vi "Periodic Tasks.vi"(8 "error in":errorcluster) -> ()   [LabVIEW 2016]
doc: "This VI runs in parallel to other tasks. It can contain as many user-defined periodic loops as you need. These can carry out PID or other sorts of timed response."
uses:
  <vilib>/Rock Robotics/WPI/Utilities/WPI_GetSetVariantRefNum.vi
panel:
  out "Object 2":T1
  out "Data Out":u8[](array[numeric])
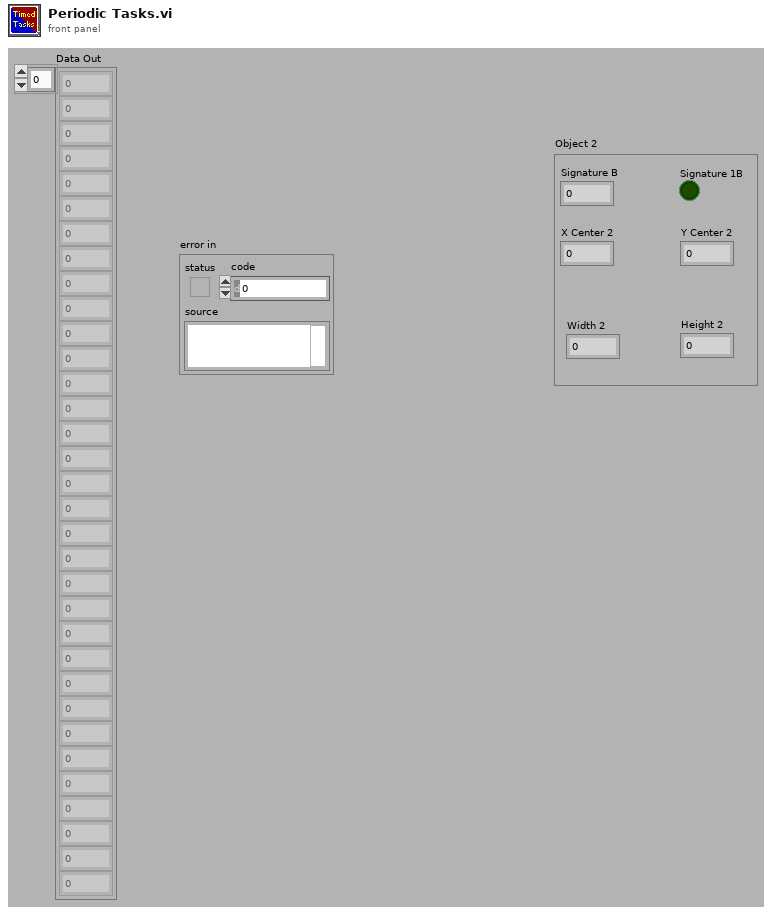
[diagram p1: front panel]
types:
  T1 = cluster{"Signature B":dbl, "Signature 1B":bool, "X Center 2":dbl, "Y Center 2":dbl, "Width 2":dbl, "Height 2":dbl}
  T2 = typedef "WPI_I2CDevRef.ctl" = cluster{"DevStatus":errorcluster, "Device Address":u8, "Handle":i32, "I2C Bus":T3}
  T3 = typedef "i2c_bus.ctl" = enum16{"I2C On-Board", "I2C MXP", "Invalid"}
  T4 = typedef "WPI_JoystickDevRef.ctl" = cluster{"Device":T5}
  T5 = typedef "WPI_JoystickDeviceEnum.ctl" = enum16{"USB 0", "USB 1", "USB 2", "USB 3", "USB 4", "USB 5"}
  T6 = typedef "WPI_MotorControlDeviceRef.ctl" = cluster{"DeviceStatus":errorcluster, "Type":T7, "PWM":cluster{"PWM Channel":T8, "DeadBand":T9}, "CAN":cluster{"Device Number":u8, "SetOutput VI Ref":variant, "GetOutput VI Ref":variant, "Enable VI Ref":variant, "Disable VI Ref":variant, "Data":variant}, "Invert":bool}
  T7 = typedef "WPI_MotorControlType.ctl" = enum16{"PWM", "CAN"}
  T8 = typedef "FPGA_DIOPWMChannel.ctl" = enum8{"PWM 0", "PWM 1", "PWM 2", "PWM 3", "PWM 4", "PWM 5", "PWM 6", "PWM 7", "PWM 8", "PWM 9", "PWM MXP 0", "PWM MXP 1", "PWM MXP 2", "PWM MXP 3", "PWM MXP 4", "PWM MXP 5", "PWM MXP 6", "PWM MXP 7", "PWM MXP 8", "PWM MXP 9", "Invalid"}
  T9 = typedef "WPI_PWMDeadband.ctl" = cluster{"Name":string, "maxPositivePwm":i32, "minPositivePwm":i32, "centerPwm":i32, "maxNegativePwm":i32, "minNegativePwm":i32, "angularRange":u16}
  T10 = cluster{"Height":dbl, "Signature A":dbl, "Signature 1A":bool, "X Center":dbl, "Y Center":dbl, "Width":dbl}
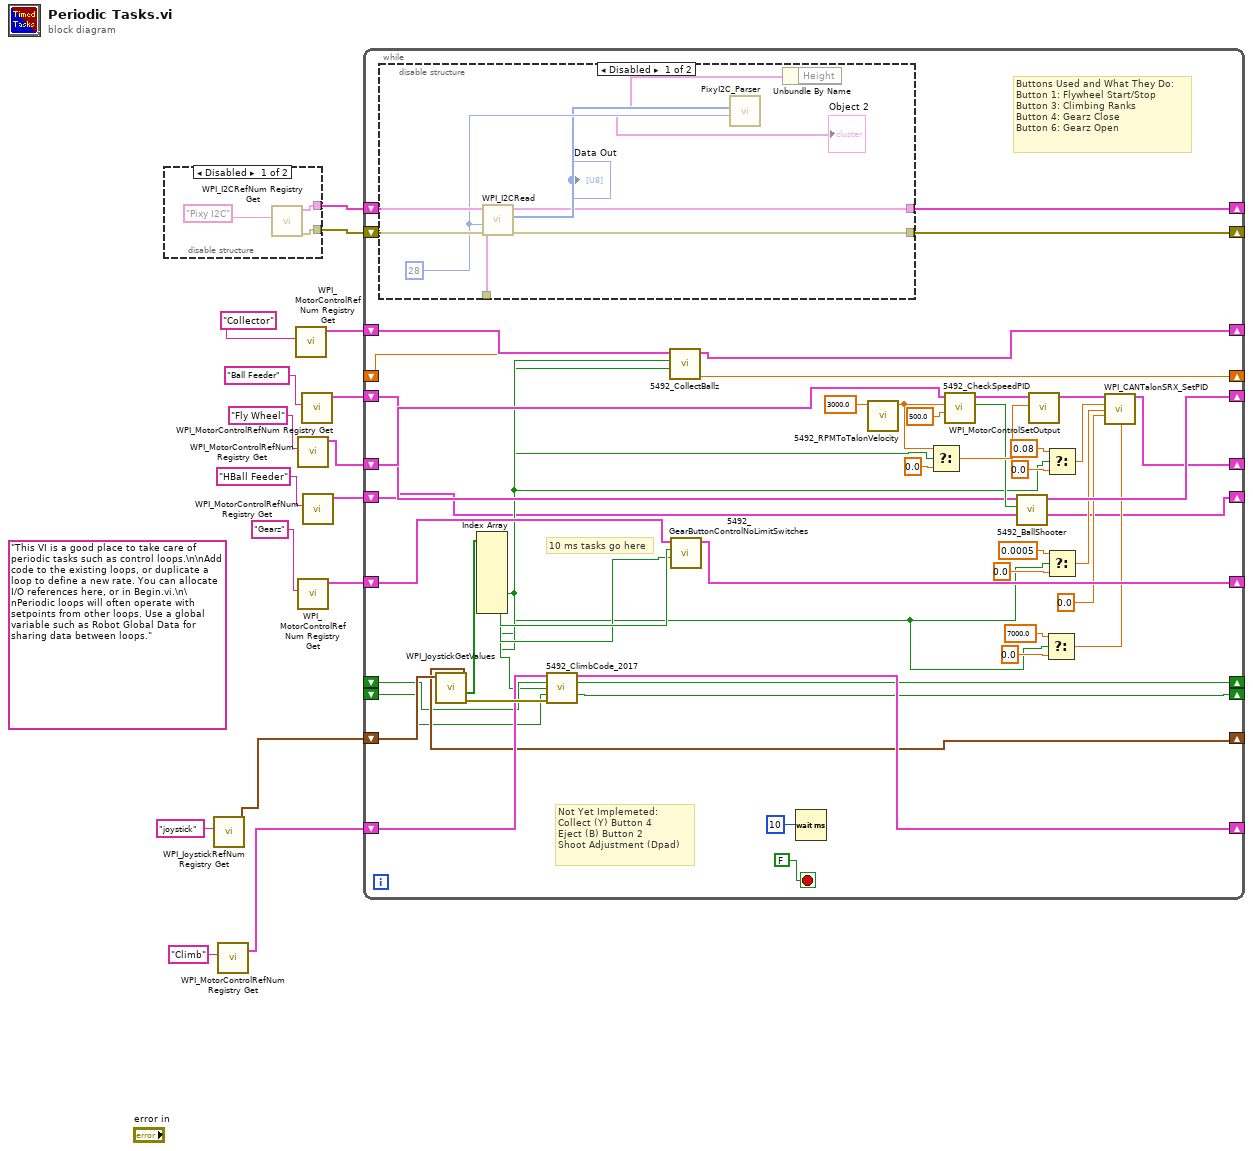
[diagram p0: block diagram]
diagram:
  (unwired) "This VI is a good place to take care of periodic tasks such as control loops.\n\nAdd code to the existing loops, or duplicate a loop to define a new rate. You can allocate I/O references here, or in Begin.vi.\n\nPeriodic loops will often operate with setpoints from other loops. Use a global variable such as Robot Global Data for sharing data between loops."
  n1 = disable-structure shown="Disabled" {
    disable-tunnel: [w18 _] -> w6
    disable-tunnel: [w17 _] -> w5
    frame Disabled {
      n2 = call <vilib>:"WPI_I2CRefNum Registry Get.vi"("refnum name"="Pixy I2C") -> ("error out"=w17:errorcluster, "I2CDevRef"=w18:T2)  [unwired: 9 in]
    }
    frame Enabled {
    }
  }
  n3 = call <vilib>:"WPI_JoystickRefNum Registry Get.vi"("refnum name"="joystick") -> ("JoystickDevRef"=w14:T4)  [unwired: 9 in, 1 out]
  n4 = call <vilib>:"WPI_MotorControlRefNum Registry Get.vi"("refnum name"="Climb") -> ("MotorControlDevRef"=w13:T6)  [unwired: 9 in, 1 out]
  n5 = call <vilib>:"WPI_MotorControlRefNum Registry Get.vi"("refnum name"="Collector") -> ("MotorControlDevRef"=w3:T6)  [unwired: 9 in, 1 out]
  n6 = call <vilib>:"WPI_MotorControlRefNum Registry Get.vi"("refnum name"="Fly Wheel") -> ("MotorControlDevRef"=w9:T6)  [unwired: 9 in, 1 out]
  n7 = call <vilib>:"WPI_MotorControlRefNum Registry Get.vi"("refnum name"="Gearz") -> ("MotorControlDevRef"=w11:T6)  [unwired: 9 in, 1 out]
  n8 = call <vilib>:"WPI_MotorControlRefNum Registry Get.vi"("refnum name"="Ball Feeder") -> ("MotorControlDevRef"=w7:T6)  [unwired: 9 in, 1 out]
  n9 = call <vilib>:"WPI_MotorControlRefNum Registry Get.vi"("refnum name"="HBall Feeder") -> ("MotorControlDevRef"=w1:T6)  [unwired: 9 in, 1 out]
  n10 = while {
    shift-right: [w65] -> _
    shift-left: w13 -> [w66]
    shift-right: [w64] -> _
    shift-left: w14 -> [w69]
    shift-right: [w62] -> _
    shift-left: w11 -> [w63]
    shift-right: [w39] -> _
    shift-left: w9 -> [w60]
    shift-right: [w53] -> _
    shift-left: w7 -> [w54]
    shift-right: [w52] -> _
    shift-left: _ -> [w51]
    shift-right: [w50] -> _
    shift-left: _ -> [w49]
    shift-right: [w45] -> _
    shift-left: w5 -> [w47]
    shift-right: [w46] -> _
    shift-left: w6 -> [w48]
    shift-right: [w37] -> _
    shift-left: w3 -> [w38]
    shift-right: [w34] -> _
    shift-left: _ -> [w33]
    shift-right: [w20] -> _
    shift-left: w1 -> [w21]
    stop <- FALSE stop-if-true
    # "Not Yet Implemeted:\nCollect (Y) Button 4\nEject (B) Button 2\nShoot Adjustment (Dpad)"
    # "Buttons Used and What They Do:\nButton 1: Flywheel Start/Stop\nButton 3: Climbing Ranks\nButton 4: Gearz Close\nButton 6: Gearz Open"
    # "10 ms tasks go here"
    n11 = disable-structure shown="Disabled" {
      disable-tunnel: w48 -> [w76 _]
      disable-tunnel: w47 -> [w75 _]
      disable-tunnel: [w74 _] -> w46
      disable-tunnel: [w73 _] -> w45
      frame Disabled {
        w79 = u8 28 ("I2CBytesToRead")
        n12 = call <vilib>:"WPI_I2CRead.vi"("error in (no error)"=w75, "I2CBytesToRead"=w79, "I2CDevRef"=w76) -> ("error out"=w73:errorcluster, "Data Out"=w78:u8[], "I2CDevRef"=w74:T2)  [unwired: 6 in]
        "Data Out" <- w78
        n13 = call "PixyI2C_Parser.vi"("Array Size"=w79, "Array"=w78) -> ("Object 2"=→"Object 2":T1, "Object 1"=w72:T10)  [unwired: 7 in]
        n14 = Unbundle By Name(w72) -> ()  [unwired: 1 out]
      }
      frame Enabled {
      }
    }
    n15 = call <vilib>:"WPI_JoystickGetValues.vi"("JoystickDevRef"=w69) -> ("error out"=w67:errorcluster, "Buttons"=w68:bool[], "JoystickDevRef"=w64:T4)  [unwired: 6 in, 2 out]
    n16 = Index Array(array=w68) -> (element #1=w44:bool, element #2=w35:bool, element #3=w43:bool, element #4=w36:bool, element #5=w42:bool, element #6=w29:bool)  [unwired: 8 in, 2 out]
    n17 = call "5492_ClimbCode_2017.vi"("MotorControlDevRef"=w66, "Stuck? (Input)"=w51, "Button Press"=w42, "Rope Grabbed? (Input)"=w49, "error in (no error)"=w67) -> ("MotorControlDevRef"=w65:T6, "Stuck? (Output)"=w52:bool, "Rope Grabbed? (Output)"=w50:bool)  [unwired: 7 in, 1 out]
    n18 = call "5492_CollectBallz.vi"("Current Collect"=w33, "Reject Ballz"=w35, "Collect Ballz"=w36, "MotorControlDevRef"=w38) -> ("Current Collect"=w34:dbl, "MotorControlDevRef"=w37:T6)  [unwired: 6 in]
    n19 = call "5492_GearButtonControlNoLimitSwitches.vi"("Button (Close)"=w43, "Button (Open)"=w44, "MotorControlDevRef"=w63) -> ("MotorControlDevRef"=w62:T6)  [unwired: 8 in]
    n20 = Wait (ms)(milliseconds to wait=u32 10) -> ()  [unwired: 1 out]
    n21 = call "5492_RPMToTalonVelocity.vi"("RPM"=3000.0) -> ("Talon Velocity"=w56:dbl)  [unwired: 10 in]
    n22 = Select(t=w56, s=w29, f=0.0) -> (s? t:f=w58:dbl)
    n23 = call "5492_CheckSpeedPID.vi"("Margin Of Error"=500.0, "Goal"=w56, "CAN Talon SRX Ref In"=w60) -> ("Speed Reached"=w55:bool, "CAN Talon SRX Ref In Out"=w59:T6)  [unwired: 6 in]
    n24 = call "5492_BallShooter.vi"("MotorControlDevRef Horizontal"=w21, "Shoot?"=w55, "MotorControlDevRef In"=w54) -> ("MotorControlDevRef Horizontal Out"=w20:T6, "MotorControlDevRef Out"=w53:T6)  [unwired: 7 in]
    n25 = call <vilib>:"WPI_MotorControlSetOutput.vi"("Output"=w58, "MotorControlDevRef"=w59) -> ("MotorControlDevRef"=w40:T6)  [unwired: 7 in, 2 out]
    n26 = Select(t=7000.0, s=w29, f=0.0) -> (s? t:f=w25:dbl)
    n27 = Select(t=0.08 ("f"), s=w29, f=0.0) -> (s? t:f=w28:dbl)
    n28 = Select(t=0.0005 ("f"), s=w29, f=0.0) -> (s? t:f=w27:dbl)
    n29 = call <vilib>:"WPI_CANTalonSRX_SetPID.vi"("CAN Talon SRX Ref"=w40, "P"=w28, "I"=w27, "D"=0.0 ("f"), "I Zone"=w25) -> ("CAN Talon SRX Ref"=w39:T6)  [unwired: 9 in, 1 out]
  }
